vi "Run.vi"(8 "error in (no error)":errorcluster, 11 "MB in":refnum<class "Master CR.lvclass">) -> (0 "error out":errorcluster, 3 "MB out":refnum<class "Master CR.lvclass">)   [LabVIEW 2021, in "Master CR.lvclass"]
uses:
  Master CR.lvclass
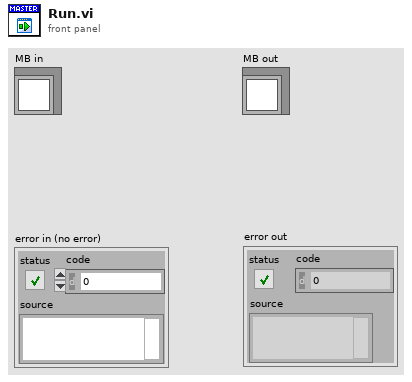
[diagram p1: front panel]
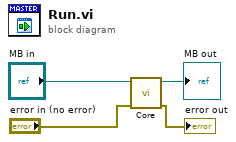
[diagram p0: block diagram]
diagram:
  n1 = call-dynamic "Core.vi"("error in (no error)"="error in (no error)", "MB in"="MB in") -> ("consumer error"=→"error out":errorcluster, "MB out"=→"MB out":refnum<class "Master CR.lvclass">)  [unwired: 8 in]
